vi "Set Handling Error.vi"(8 "error in (no error)":errorcluster, 9 "Error":errorcluster, 10 "Error Level":T1, 11 "Elevator Controller in":refnum<class "Elevator Controller.lvclass">) -> (0 "error out":errorcluster, 3 "Elevator Controller out":refnum<class "Elevator Controller.lvclass">)   [LabVIEW 2019, in "Elevator Controller.lvlib" / "Elevator Controller.lvclass"]
uses:
  Elevator Controller.lvclass
  Error Level -enum.ctl
  Error Data.ctl
  Elevator Controller Messages/Set State Msg/Set State Msg.lvclass
  State -Enum.ctl
  <vilib>/ActorFramework/Actor/Actor.lvclass
  C:/Program Files (x86)/National Instruments/LabVIEW 2019/vi.lib/ActorFramework/Actor/Actor.lvclass
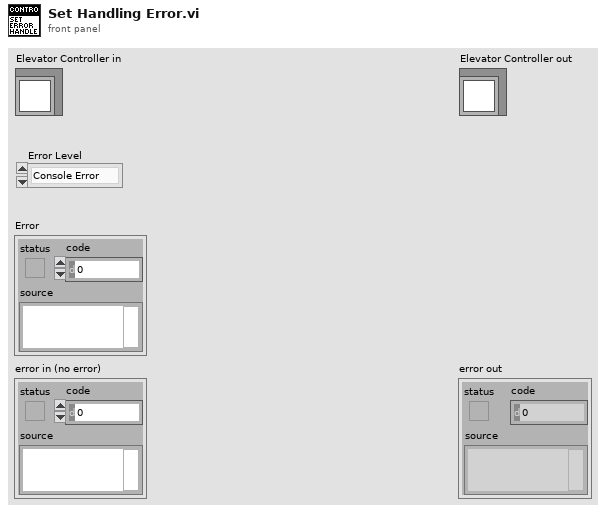
[diagram p1: front panel]
types:
  T1 = typedef "Elevator Controller.lvlib/Elevator Controller.lvclass/Error Level -enum.ctl" = enum16{"Console Error", "Sensor Interface IO Error", "Process Step Error"}
  T2 = typedef "Elevator Controller.lvlib/Elevator Controller.lvclass/Error Data.ctl" = cluster{"Description":string, "Error Level":T1, "Time Stamp":timestamp}
  T3 = typedef "Elevator Controller.lvlib/Elevator Controller.lvclass/State -Enum.ctl" = enum16{"Initial", "Wait for First Request", "Start and Move", "Analysis", "Continue Travel", "Stop at Floor", "Open and Close Door Sequence", "No request Remaining", "Emergency Call", "Terminate Process"}
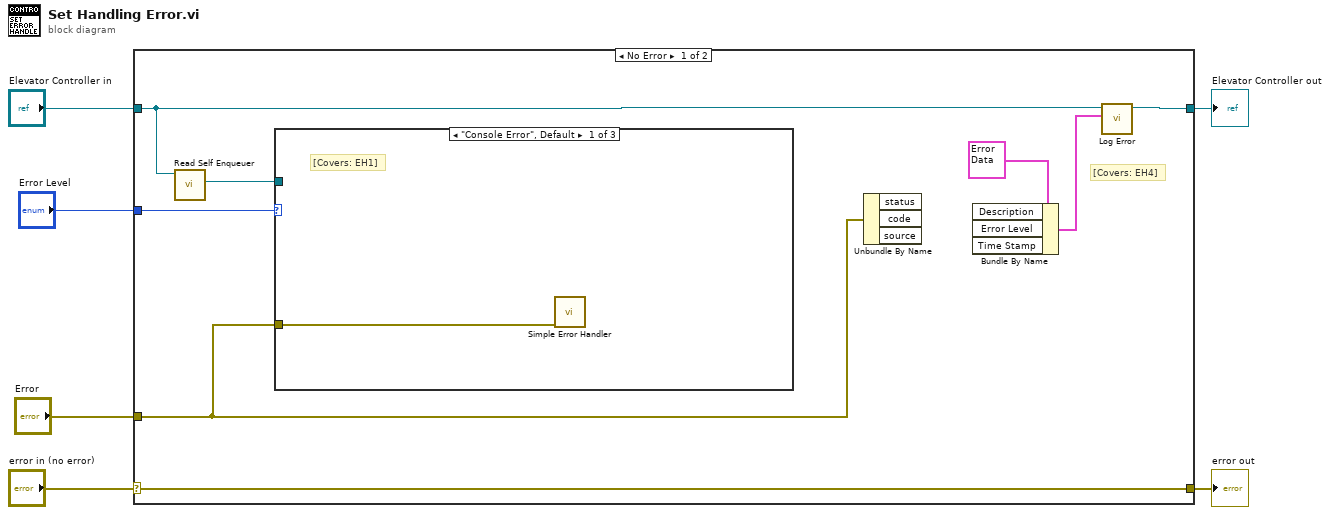
[diagram p0: block diagram]
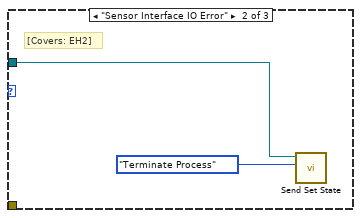
[diagram p2: hidden frame]
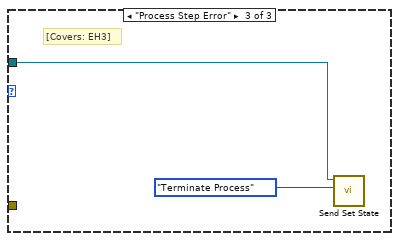
[diagram p3: hidden frame]
diagram:
  n1 = case shown="No Error" "error in (no error)" {
    selector: "error in (no error)" -> [w14 w21]
    tunnel: [w14 w21] -> w5
    tunnel: [w12 w20] -> w3
    tunnel: "Elevator Controller in" -> [w9 w20]
    tunnel: "Error Level" -> [w13 _]
    tunnel: "Error" -> [w7 _]
    frame No Error {
      # "[Covers: EH4]"
      n2 = call <vilib>:"Read Self Enqueuer.vi"("Actor"=w9) -> ("Self Enqueuer"=w8:refnum<class "Message Enqueuer.lvclass">)  [unwired: 10 in]
      n3 = case shown="\"Console Error\", Default" w13 {
        tunnel: w8 -> [_ w16 w18]
        tunnel: w7 -> [w15 _ _]
        frame "Console Error", Default {
          # "[Covers: EH1]"
          n4 = call <vilib>:"Simple Error Handler.vi"("error in (no error)"=w15) -> ()  [unwired: 4 in, 5 out]
        }
        frame "Sensor Interface IO Error" {
          # "[Covers: EH2]"
          n5 = call "Send Set State.vi"("State"=State_-Enum."Terminate Process", "Message Enqueuer"=w16) -> ()  [unwired: 8 in, 2 out]
        }
        frame "Process Step Error" {
          # "[Covers: EH3]"
          n6 = call "Send Set State.vi"("State"=State_-Enum."Terminate Process", "Message Enqueuer"=w18) -> ()  [unwired: 8 in, 2 out]
        }
      }
      n7 = Unbundle By Name(w7) -> ()  [unwired: 3 out]
      n8 = Bundle By Name(cluster=T2 {"Description"="", "Error Level"=enum."Console Error", "Time Stamp"=timestamp(0 s since 1904-01-01)} ("Error Data")) -> (w10:T2)  [unwired: 3 in]
      n9 = call "Log Error.vi"("Error Data"=w10, "Elevator Controller in"=w9) -> ("Elevator Controller out"=w12:refnum<class "Elevator Controller.lvclass">)  [unwired: 8 in, 1 out]
    }
    frame Error {
    }
  }
  "error out" <- w5
  "Elevator Controller out" <- w3
